vi "aim green.vi"(8 "error in (no error)":errorcluster, 11 "KNR in":T1) -> (0 "error out":errorcluster, 2 "Boolean":bool=TRUE, 3 "KNR out":T1, 4 "DC Position Offset":i32)   [LabVIEW 2013]
uses:
  <userlib>/KNR OS 3.0 LabVIEW Toolkit/Type Definition/KNR3 Reference.ctl
  <userlib>/_FPGA Interface Advanced Tools/FPGA Interface Base/FPGA Interface Base.lvclass
  <userlib>/KNR OS 3.0 LabVIEW Toolkit/Type Definition/Resource.ctl
  Global 1.vi
panel:
  out "Aim":dbl
  out "e pix":dbl
  out "CM":dbl
  in  "STOP":bool
  out "Error(deg)":ext
  out "中心坐标与对应的面积":dbl[][](array[numeric])
  out "处理后":T3(plugin-control)
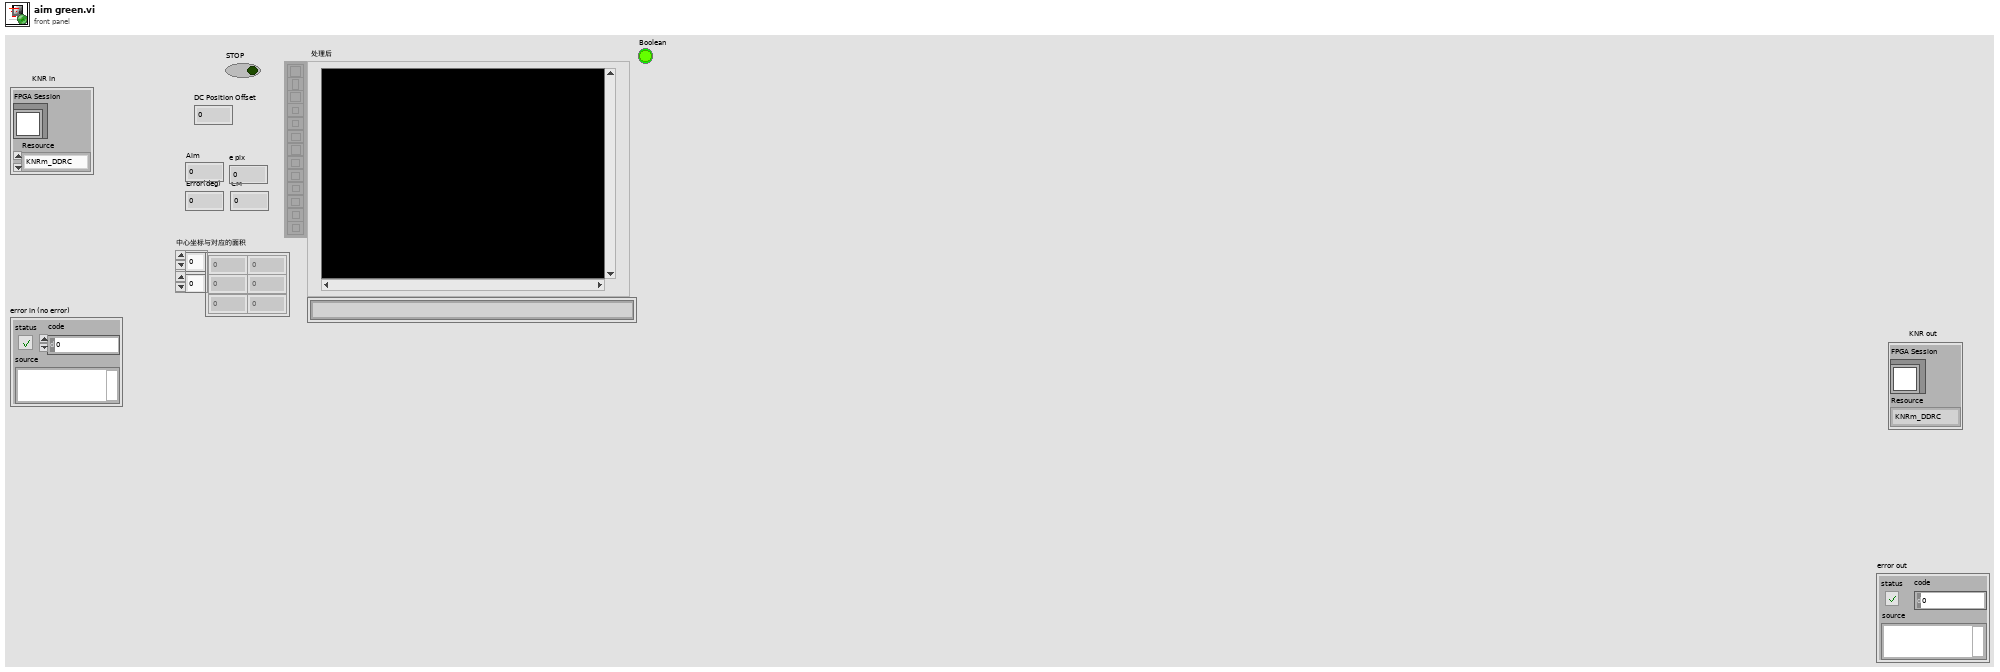
[diagram p1: front panel]
types:
  T1 = typedef "KNR3 Reference.ctl" = cluster{"FPGA Session":refnum<class "FPGA Interface Base.lvclass">, "Resource":T2}
  T2 = typedef "Resource.ctl" = enum16{"KNRm_DDRC", "KNRm_DDDD", "KNRm_DDDR", "KNRm_DDDC", "KNR"}
  T3 = typedef "IMAQ Image.ctl" = refnum<image>
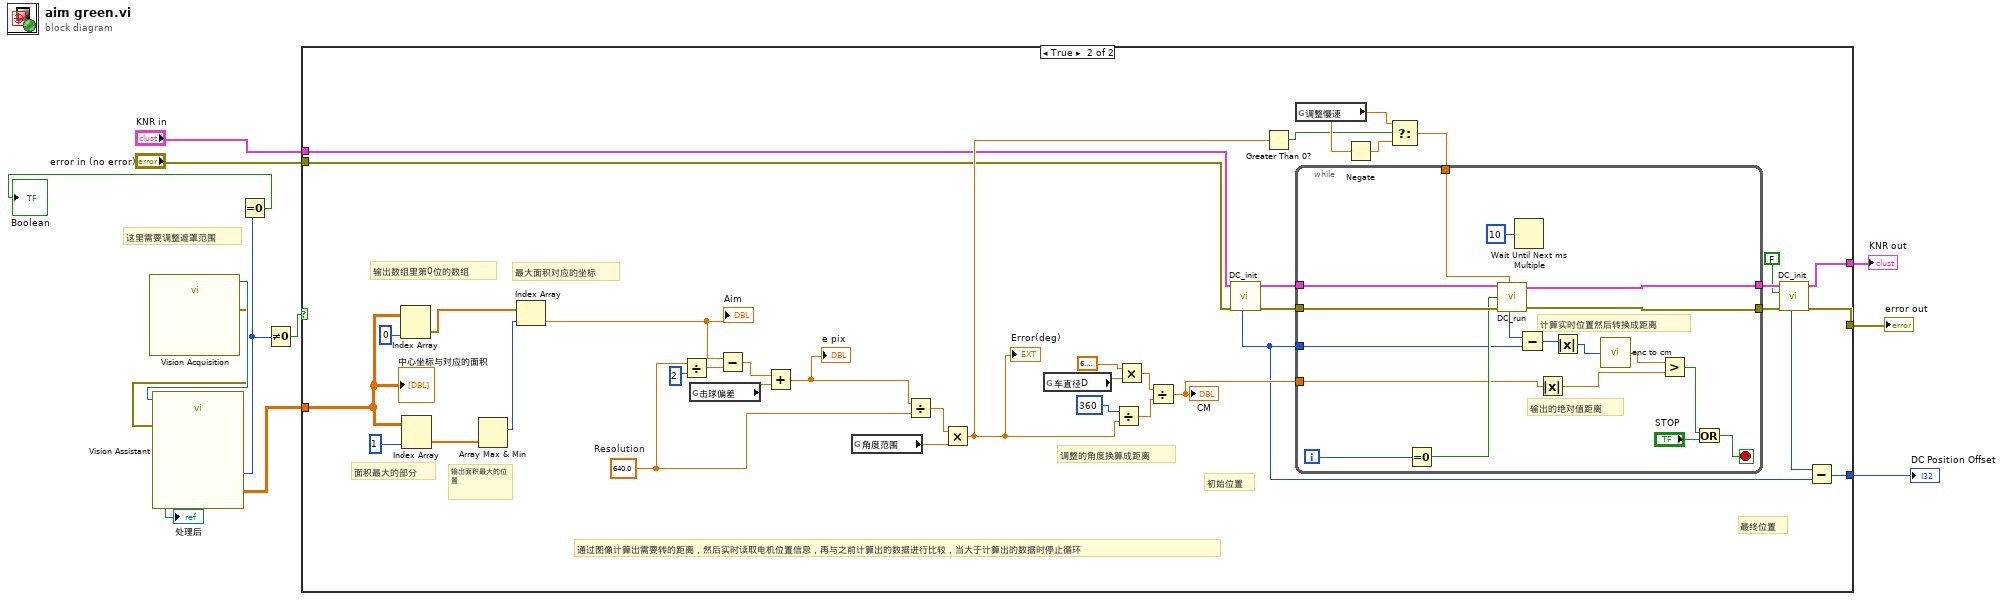
[diagram p0: block diagram]
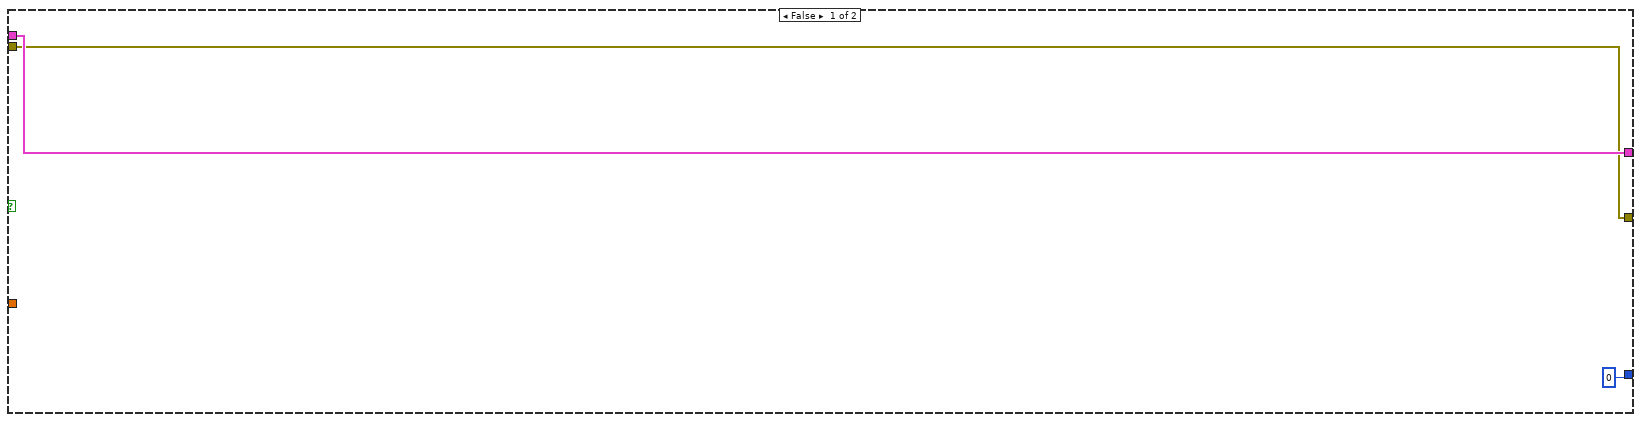
[diagram p2: hidden frame]
diagram:
  # "这里需要调整遮罩范围"
  n1 = call "Vision Acquisition"() -> ("Image Out"=w5:T3, "error out"=w3:errorcluster)  [unwired: 26 in]
  n2 = call "Vision Assistant"("Image In"=w5, "error in"=w3) -> ("Image Out"=→"处理后":T3, "Number of Particles (coordinate)"=w2:i32, "Particle Measurements (Pixels) (coordinate)"=w4:dbl[][])  [unwired: 22 in, 1 out]
  n3 = Equal To 0?(x=w2) -> (x = 0?=→"Boolean":bool)
  n4 = Not Equal To 0?(x=w2) -> (x != 0?=w8:bool)
  n5 = case shown="True" w8 {
    tunnel: [w15 w27] -> w12
    tunnel: [w14 w26] -> w11
    tunnel: w4 -> [_ w20]
    tunnel: [0 w18] -> w9
    tunnel: "KNR in" -> [w15 w17]
    tunnel: "error in (no error)" -> [w14 w16]
    frame False {
    }
    frame True {
      w37 = 640.0  # Resolution
      # "最终位置"
      # "最大面积对应的坐标"
      # "面积最大的部分"
      # "输出面积最大的位置"
      # "输出数组里第0位的数组"
      # "调整的角度换算成距离"
      # "初始位置"
      # "通过图像计算出需要转的距离，然后实时读取电机位置信息，再与之前计算出的数据进行比较，当大于计算出的数据时停止循环"
      n6 = Index Array(array=w20, index (col)=0 ("disabled index (col)")) -> (element=w23:dbl[])  [unwired: 1 in]
      n7 = Index Array(array=w20, index (col)=1 ("disabled index (col)")) -> (element=w22:dbl[])  [unwired: 1 in]
      n8 = Array Max & Min(array=w22) -> (max index (indices)=w21:i32)  [unwired: 3 out]
      n9 = Index Array(array=w23, index=w21) -> (element=w19:dbl)
      "Aim" <- w19
      n10 = Divide(x=w37, y=2) -> (x/y=w36:dbl)
      n11 = global read "Global 1.vi" "击球偏差"() -> (w52:dbl)
      n12 = Subtract(x=w19, y=w36) -> (x-y=w53:dbl)
      n13 = Add(x=w53, y=w52) -> (x+y=w49:dbl)
      "e pix" <- w49
      n14 = global read "Global 1.vi" "角度范围"() -> (w51:dbl)
      n15 = Divide(x=w49, y=w37) -> (x/y=w50:dbl)
      n16 = Multiply(x=w50, y=w51) -> (x*y=w30:dbl)
      "Error(deg)" <- w30
      n17 = global read "Global 1.vi" "车直径D"() -> (w46:dbl)
      n18 = Divide(x=360, y=w30) -> (x/y=w44:dbl)
      n19 = Multiply(x=6.283185307179586, y=w46) -> (x*y=w45:dbl)
      n20 = Divide(x=w45, y=w44) -> (x/y=w41:dbl)
      "CM" <- w41
      n21 = call "DC_init.vi"("error in (no error)"=w16, "KNR in"=w17) -> ("error out"=w42:errorcluster, "KNR out"=w43:T1, "output\nPosition_1"=w34:i32)  [unwired: 6 in, 1 out]
      n22 = Greater Than 0?(x=w30) -> (x > 0?=w31:bool)
      n23 = global read "Global 1.vi" "调整慢速"() -> (w32:dbl)
      n24 = Negate(x=w32) -> (-x=w33:dbl)
      n25 = Select(t=w32, s=w31, f=w33) -> (s? t:f=w29:dbl)
      n26 = while {
        tunnel: w43 -> [w71]
        tunnel: w42 -> [w70]
        tunnel: [w69] -> w40
        tunnel: [w68] -> w39
        tunnel: w41 -> [w59]
        tunnel: w34 -> [w56]
        tunnel: w29 -> [w54]
        i -> [w62]
        stop <- w65 stop-if-true
        # "输出的绝对值距离"
        # "计算实时位置然后转换成距离"
        n27 = Equal To 0?(x=w62) -> (x = 0?=w61:bool)
        n28 = call "DC_run.vi"("KNR in"=w71, "speed_1"=w54, "reinitialize? (F)"=w61, "error in (no error)"=w70) -> ("Position_1"=w55:i32, "KNR out"=w69:T1, "error out"=w68:errorcluster)  [unwired: 2 in, 1 out]
        n29 = Wait Until Next ms Multiple(millisecond multiple=u32 10) -> ()  [unwired: 1 out]
        n30 = Subtract(x=w55, y=w56) -> (x-y=w67:i32)
        n31 = Absolute Value(x=w59) -> (abs(x)=w66:dbl)
        n32 = Absolute Value(x=w67) -> (abs(x)=w58:i32)
        n33 = call "enc to cm.vi"("E"=w58) -> ("CM"=w57:dbl)  [unwired: 1 in]
        n34 = Greater?(x=w57, y=w66) -> (0:w64:bool)
        n35 = Or(x=w64, y="STOP") -> (x .or. y?=w65:bool)
      }
      n36 = call "DC_init.vi"("error in (no error)"=w39, "Enable Motor(T)"=FALSE, "KNR in"=w40) -> ("error out"=w26:errorcluster, "KNR out"=w27:T1, "output\nPosition_1"=w28:i32)  [unwired: 5 in, 1 out]
      n37 = Subtract(x=w28, y=w34) -> (x-y=w18:i32)
      "中心坐标与对应的面积" <- w20
    }
  }
  "error out" <- w11
  "KNR out" <- w12
  "DC Position Offset" <- w9
